vi "Get-client-channels-by-type.vi"(8 "error in (no error)":errorcluster, 10 "Module type":T1=enum."Server", 11 "ModComm in":T2) -> (0 "error out":errorcluster, 2 "Client channels":refnum<queue>[](array[refnum]), 3 "ModComm out":T2)   [LabVIEW 2013, in "SLMServer.lvlib" / "SLMServer.lvclass"]
uses:
  SLMServer.lvclass
  Object-reference.ctl
  Supported-module-types.ctl
  SA-SLMAPI/Sources/Message.lvclass
  SLMServer.lvclass/SLMServer.ctl
  Read Clients.vi
  Read Client channels.vi
  Read Server channel.vi
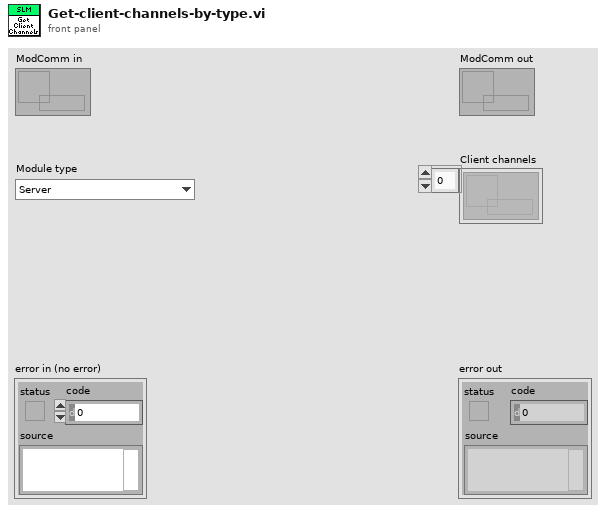
[diagram p1: front panel]
types:
  T1 = typedef "SLMServer.lvlib/SLMServer.lvclass/Supported-module-types.ctl" = enum16{"SLMControl", "PowderDeposition", "CameraVision", "Server", "All", "StrategyParser", "MaterialCharacterization", "StatusMonitor", "SLMSimulation", "LaserCharacterization"}
  T2 = typedef "SLMServer.lvlib/SLMServer.lvclass/Object-reference.ctl" = refnum<data-value>
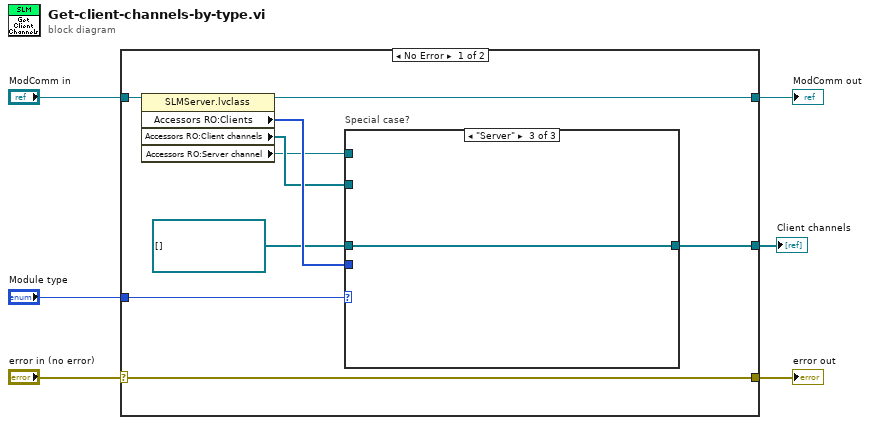
[diagram p0: block diagram]
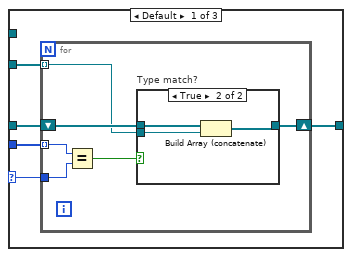
[diagram p2: hidden frame]
diagram:
  n1 = case shown="No Error" "error in (no error)" {
    selector: "error in (no error)" -> [w15 w34]
    tunnel: [w15 w34] -> w5
    tunnel: [w13 w33] -> w3
    tunnel: "ModComm in" -> [w14 w33]
    tunnel: "Module type" -> [w8 _]
    tunnel: [w11 _] -> w1
    frame No Error {
      n2 = property class="SLMServer.lvclass"(reference=w14) -> (reference out=w13:T2, "Accessors RO:Clients"=w12:T1[], "Accessors RO:Client channels"=w10:refnum<queue>[], "Accessors RO:Server channel"=w9:refnum<queue>)  [unwired: 1 in, 1 out]
      n3 = case "Special case?" shown="\"Server\"" w8 {
        selector: w8 -> [w16 _ _]
        tunnel: w12 -> [w20 _ _]
        tunnel: [w19 w31 w32] -> w11
        tunnel: refnum<queue>[] [] -> [w18 _ w32]
        tunnel: w10 -> [w17 w31 _]
        tunnel: w9 -> [_ _ _]
        frame Default {
          n4 = for {
            tunnel: w20 -> [w25] mode=indexing
            tunnel: w16 -> [w26]
            shift-right: [w21] -> w19
            shift-left: w18 -> [w24]
            tunnel: w17 -> [w22] mode=indexing
            n5 = Equal?(x=w25, y=w26) -> (x = y?=w23:bool)
            n6 = case "Type match?" shown="True" w23 {
              tunnel: w24 -> [w27 w30]
              tunnel: w22 -> [_ w29]
              tunnel: [w27 w28] -> w21
              frame False {
              }
              frame True {
                n7 = Build Array (concatenate)(w30, w29) -> (w28:refnum<queue>[])
              }
            }
          }
        }
        frame "All" {
        }
        frame "Server" {
        }
      }
    }
    frame Error {
    }
  }
  "error out" <- w5
  "ModComm out" <- w3
  "Client channels" <- w1
